vi "ProjectLoader.vi"() -> ()   [LabVIEW 2014]
uses:
  <resource>/Framework/Providers/API/ItemRef.ctl
  GCMCore/Providers/Veritech_GCM/Support/Framework/ItemSelection/ItemSelection.lvlib
panel:
  out "Type String":string
  out "Type GUID":string
  in  "stop":bool
  in  "Tree":string(tree)
  in  "Path":path=path "E:/Projects/8205/Trunk/Tests/TestProject/GcodeManagerTestProject.lvproj"
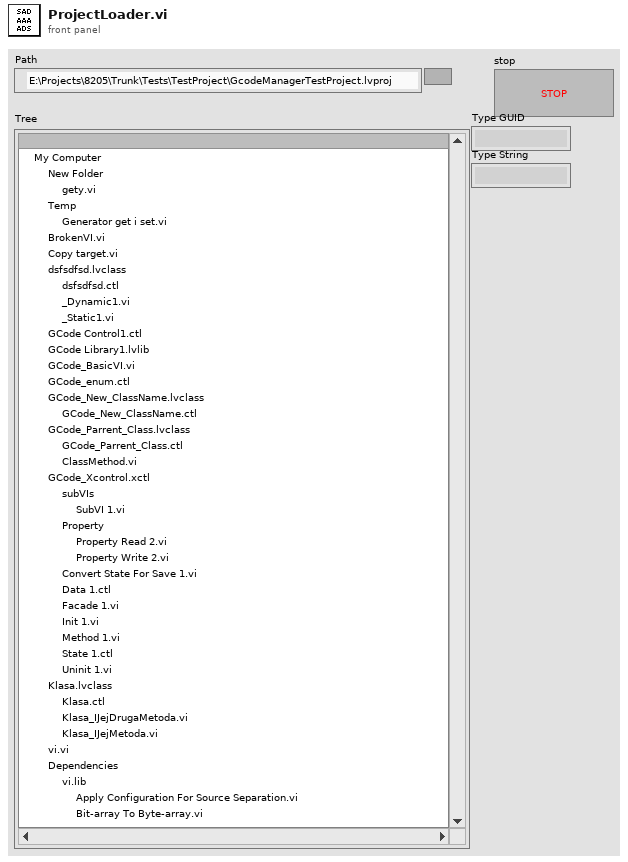
[diagram p1: front panel]
types:
  T1 = typedef "ItemRef.ctl" = u64
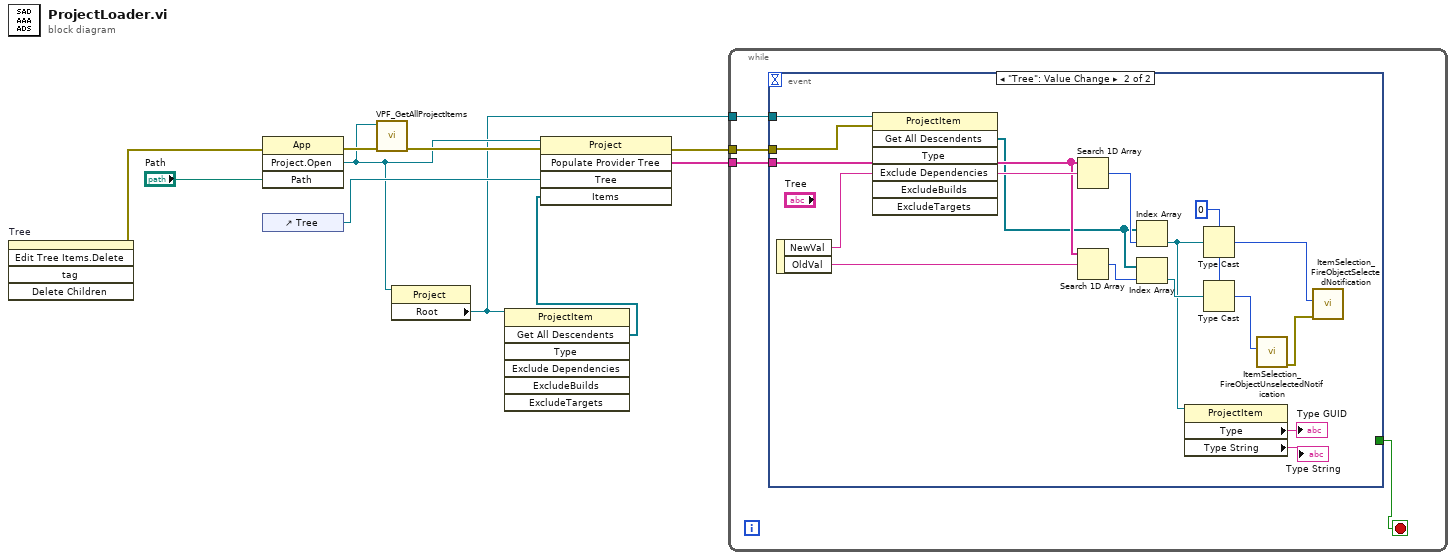
[diagram p0: block diagram]
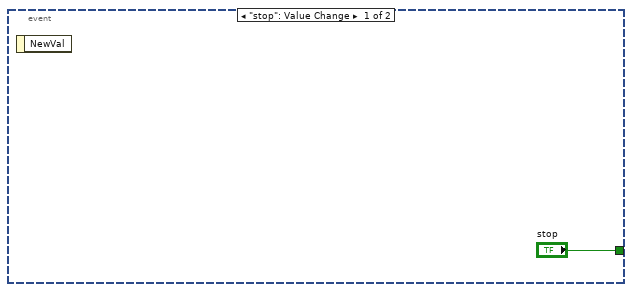
[diagram p2: hidden frame]
diagram:
  n1 = invoke on="Tree" class="Tree (strict)" method="Edit Tree Items.Delete"() -> (error out=w4:errorcluster)  [unwired: 5 in, 4 out]
  n2 = invoke class="App" method="Project.Open"(error in=w4, "Path"="Path") -> (error out=w6:errorcluster, "Project:Open"=w3:refnum<vi>)  [unwired: 2 in, 2 out]
  n3 = control-ref of="Tree"() -> (w9:refnum<vi>)
  n4 = call <resource>:"VPF_GetAllProjectItems.vi"("error in (no error)"=w6, "ProjectRefNum"=w3) -> ("error out"=w5:errorcluster)  [unwired: 5 in, 4 out]
  n5 = property class="Project"(reference=w3) -> ("Root"=w1:refnum<vi>)  [unwired: 1 in, 2 out]
  n6 = invoke class="ProjectItem" method="Get All Descendents"(reference=w1) -> ("All Descendents"=w2:refnum<vi>[])  [unwired: 6 in, 6 out]
  n7 = invoke class="Project" method="Populate Provider Tree"(reference=w3, error in=w5, "Tree"=w9, "Items"=w2) -> (error out=w8:errorcluster, "Populate Provider Tree"=w7:string[])  [unwired: 1 in, 3 out]
  n8 = while {
    tunnel: w8 -> [w13]
    tunnel: w7 -> [w12]
    tunnel: w1 -> [w11]
    stop <- w14 stop-if-true
    n9 = event shown="[1] \"Tree\": Value Change" {
      selector: _ -> [_ _]
      dyn-events: _ -> [_ _]
      timeout: _ -> [_ _]
      tunnel: ["stop" _] -> w14
      tunnel: w13 -> [_ w21]
      tunnel: w12 -> [_ w28]
      tunnel: w11 -> [_ w20]
      event "stop": Value Change {
        n10 = event-data() -> ()  [unwired: 1 in, 1 out]
      }
      event "Tree": Value Change {
        w25 = T1 0 ("Object")
        n11 = event-data() -> ("NewVal"=w30:string, "OldVal"=w27:string)  [unwired: 1 in]
        n12 = invoke class="ProjectItem" method="Get All Descendents"(reference=w20, error in=w21) -> ("All Descendents"=w19:refnum<vi>[])  [unwired: 5 in, 6 out]
        n13 = Search 1D Array(1D array=w28, element=w30) -> (index of element=w31:i32)  [unwired: 1 in]
        n14 = Search 1D Array(1D array=w28, element=w27) -> (index of element=w29:i32)  [unwired: 1 in]
        n15 = Index Array(array=w19, index=w31) -> (element=w18:refnum<vi>)
        n16 = Index Array(array=w19, index=w29) -> (element=w22:refnum<vi>)
        n17 = property class="ProjectItem"(reference=w18) -> ("Type"=→"Type GUID":string, "Type String"=→"Type String":string)  [unwired: 1 in, 2 out]
        n18 = Type Cast(type=w25, x=w18) -> (*(type *) &x=w24:T1)
        n19 = Type Cast(type=w25, x=w22) -> (*(type *) &x=w23:T1)
        n20 = call "ItemSelection_FireObjectUnselectedNotification.vi"("Object"=w23) -> ("error out"=w26:errorcluster)  [unwired: 10 in]
        n21 = call "ItemSelection_FireObjectSelectedNotification.vi"("error in (no error)"=w26, "Item Ref"=w24) -> ()  [unwired: 9 in, 1 out]
      }
    }
  }
